vi "Read-Save DefaultDevice.vi"(6 "Task":enum16{"Save", "Read"}(ring)=enum."Read", 11 "Soundcard":string) -> (0 "Pref Path":path, 3 "Soundcard Out":string)   [LabVIEW 2022 SP3]
panel:
  out "text":string
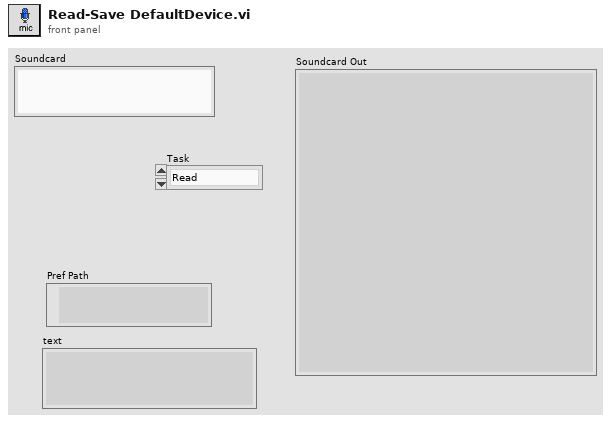
[diagram p1: front panel]
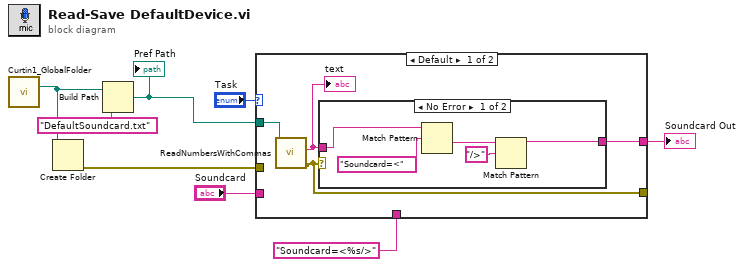
[diagram p0: block diagram]
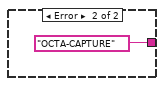
[diagram p2: hidden frame]
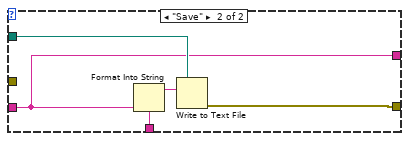
[diagram p3: hidden frame]
diagram:
  n1 = call "Curtin1_GlobalFolder.vi"() -> ("LabVIEW Data Path"=w2:path)  [unwired: 1 in, 1 out]
  n2 = Create Folder(path (use dialog)=w2) -> (error out=w3:errorcluster)  [unwired: 2 in, 2 out]
  n3 = Build Path(base path=w2, name or relative path="DefaultSoundcard.txt") -> (appended path=w7:path)
  "Pref Path" <- w7
  n4 = case shown="Default" "Task" {
    tunnel: "Soundcard" -> [_ w20]
    tunnel: w7 -> [w11 w23]
    tunnel: [w9 w21] -> _
    tunnel: [w12 w20] -> w4
    tunnel: w3 -> [_ _]
    tunnel: "Soundcard=<%s/>" ("format string") -> [_ w19]
    frame Default {
      n5 = call "ReadNumbersWithCommas.vi"("file (use dialog)"=w11) -> ("error out"=w9:errorcluster, "text"=w10:string)  [unwired: 7 in, 2 out]
      "text" <- w10
      n6 = case shown="No Error" w9 {
        tunnel: [w13 "OCTA-CAPTURE" ("Notes")] -> w12
        tunnel: w10 -> [w17 _]
        frame No Error {
          n7 = Match Pattern(string=w17, regular expression="Soundcard=<" ("format string")) -> (after substring=w16:string)  [unwired: 1 in, 3 out]
          n8 = Match Pattern(string=w16, regular expression="/>" ("format string")) -> (before substring=w13:string)  [unwired: 1 in, 3 out]
        }
        frame Error {
        }
      }
    }
    frame "Save" {
      n9 = Format Into String(format string=w19, w20) -> (resulting string=w22:string)  [unwired: 2 in, 1 out]
      n10 = Write to Text File(file (use dialog)=w23, text=w22) -> (error out=w21:errorcluster)  [unwired: 2 in, 2 out]
    }
  }
  "Soundcard Out" <- w4
